vi "Finish.vi"   [LabVIEW 2014]
doc: "This VI is called just before exiting. It is expected to close I/O refnum, save collected data, etc."
uses:
  <vilib>/Rock Robotics/WPI/Joystick/WPI_JoystickGetSetRefNum.vi
  <vilib>/Rock Robotics/WPI/RobotDrive/WPI_RobotDriveGetSetRefNum.vi
  <vilib>/Rock Robotics/WPI/Compressor/WPI_CompressorGetSetRefNum.vi
types:
  T1 = typedef "WPI_CompressorDevRef.ctl" = cluster{"DevStatus":errorcluster, "DigitalInputDevRef":T2, "RelayDevRef":T5}
  T2 = typedef "WPI_DigitalInputDevRef.ctl" = cluster{"DevStatus":errorcluster, "DIO Channel":T3, "Digital Module":T4}
  T3 = typedef "FPGA_DIOChannel.ctl" = enum8{"DIO 1", "DIO 2", "DIO 3", "DIO 4", "DIO 5", "DIO 6", "DIO 7", "DIO 8", "DIO 9", "DIO 10", "DIO 11", "DIO 12", "DIO 13", "DIO 14", "Invalid"}
  T4 = typedef "FPGA_TypedefDigitalModule.ctl" = enum16{"Digital Module 1", "Digital Module 2"}
  T5 = typedef "WPI_RelayDevRef.ctl" = cluster{"DevStatus":errorcluster, "Relay Channel":T6, "Digital Module":T4, "Relay Direction":T7}
  T6 = typedef "FPGA_DIORelayChannel.ctl" = enum8{"Relay 1", "Relay 2", "Relay 3", "Relay 4", "Relay 5", "Relay 6", "Relay 7", "Relay 8", "Invalid"}
  T7 = typedef "WPI_RelayDirection.ctl" = enum16{"Both directions", "Forward only", "Reverse only"}
  T8 = typedef "WPI_CounterDevRef.ctl" = cluster{"DevStatus":errorcluster, "CntIndex":T9}
  T9 = typedef "FPGA_CounterCtrSystemIndex.ctl" = enum8{"Ctr 0", "Ctr 1", "Ctr 2", "Ctr 3", "Ctr 4", "Ctr 5", "Ctr 6", "Ctr 7", "Invalid"}
  T10 = typedef "WPI_EncoderDevRef.ctl" = cluster{"DevStatus":errorcluster, "EncoderIndex":T11, "CounterIndex":T9, "DistancePerCount":dbl, "Decoding Type":T12}
  T11 = typedef "FPGA_EncoderIdx.ctl" = enum8{"Enc 0", "Enc 1", "Enc 2", "Enc 3", "Invalid"}
  T12 = typedef "WPI_EncoderType.ctl" = enum16{"1x", "2x", "4x"}
  T13 = typedef "WPI_RobotDriveDevRef.ctl" = cluster{"DevStatus":errorcluster, "Motors[]":T14[], "Square Inputs":bool, "Max Output":dbl}
  T14 = typedef "WPI_MotorControlDeviceRef.ctl" = cluster{"DeviceStatus":errorcluster, "Type":enum16{"PWM", "CAN"}, "PWM":cluster{"Digital Module":T4, "PWM Channel":T15, "DeadBand":T16}, "CAN":cluster{"Device Number":u8, "Control Mode":T17, "Semaphore":T18, "Max Vout":dbl}, "Invert":bool, "TransformRef":T19, "InvTransformRef":T19}
  T15 = typedef "FPGA_DIOPWMChannel.ctl" = enum8{"PWM 1", "PWM 2", "PWM 3", "PWM 4", "PWM 5", "PWM 6", "PWM 7", "PWM 8", "PWM 9", "PWM 10", "Invalid"}
  T16 = typedef "WPI_PWMDeadband.ctl" = cluster{"Name":string, "maxPositivePwm":i32, "minPositivePwm":i32, "centerPwm":i32, "maxNegativePwm":i32, "minNegativePwm":i32, "angularRange":u16}
  T17 = typedef "WPI_CANJaguar_ControlMode.ctl" = enum8{"Percent VBus", "Current", "Speed", "Position", "Voltage"}
  T18 = typedef "Semaphore RefNum" = refnum<k1>
  T19 = typedef "WPI_PWMTransform_ConPane.ctl" = refnum<vi>
  T20 = typedef "WPI_JoystickDevRef.ctl" = cluster{"Device":T21}
  T21 = typedef "WPI_JoystickDeviceEnum.ctl" = enum16{"USB 0", "USB 1", "USB 2", "USB 3", "USB 4", "USB 5"}
  T22 = typedef "WPI_SolenoidDevRef.ctl" = cluster{"DevStatus":errorcluster, "Solenoid Module":T23, "Forward Solenoid Channel":T24, "Reverse Solenoid Channel":T24}
  T23 = typedef "FPGA_TypedefSolenoidModule.ctl" = enum16{"Solenoid Module 1", "Solenoid Module 2"}
  T24 = typedef "WPI_SolenoidChannel.ctl" = enum8{"Solenoid 1", "Solenoid 2", "Solenoid 3", "Solenoid 4", "Solenoid 5", "Solenoid 6", "Solenoid 7", "Solenoid 8", "Invalid"}
  T25 = typedef "WPI_GyroDevRef.ctl" = cluster{"DevStatus":errorcluster, "Analog Module":T26, "Analog Channel":T27, "Offset":dbl, "Gain (VoltsPerDegree/Second)":dbl}
  T26 = typedef "FPGA_TypedefAnalogModule.ctl" = enum16{"Analog Module 1", "Analog Module 2"}
  T27 = typedef "FPGA_AIChannel.ctl" = enum8{"AI 1", "AI 2", "AI 3", "AI 4", "AI 5", "AI 6", "AI 7", "AI 8", "Invalid"}
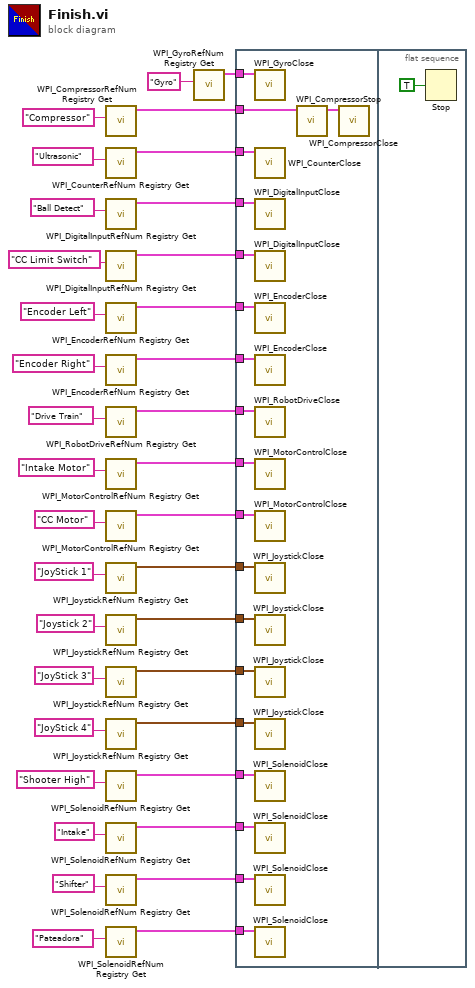
[diagram p0: block diagram]
diagram:
  n1 = call <vilib>:"WPI_CompressorRefNum Registry Get.vi"("refnum name"="Compressor") -> ("CompressorDevRef"=w31:T1)  [unwired: 9 in, 1 out]
  n2 = call <vilib>:"WPI_CounterRefNum Registry Get.vi"("refnum name"="Ultrasonic") -> ("CounterDevRef"=w6:T8)  [unwired: 9 in, 1 out]
  n3 = call <vilib>:"WPI_DigitalInputRefNum Registry Get.vi"("refnum name"="Ball Detect") -> ("DigitalInputDevRef"=w3:T2)  [unwired: 9 in, 1 out]
  n4 = call <vilib>:"WPI_DigitalInputRefNum Registry Get.vi"("refnum name"="CC Limit Switch") -> ("DigitalInputDevRef"=w30:T2)  [unwired: 9 in, 1 out]
  n5 = call <vilib>:"WPI_EncoderRefNum Registry Get.vi"("refnum name"="Encoder Left") -> ("EncoderDevRef"=w1:T10)  [unwired: 9 in, 1 out]
  n6 = call <vilib>:"WPI_EncoderRefNum Registry Get.vi"("refnum name"="Encoder Right") -> ("EncoderDevRef"=w24:T10)  [unwired: 9 in, 1 out]
  n7 = call <vilib>:"WPI_RobotDriveRefNum Registry Get.vi"("refnum name"="Drive Train") -> ("RobotDriveDevRef"=w34:T13)  [unwired: 1 in, 9 out]
  n8 = call <vilib>:"WPI_MotorControlRefNum Registry Get.vi"("refnum name"="Intake Motor") -> ("MotorControlDevRef"=w27:T14)  [unwired: 9 in, 1 out]
  n9 = call <vilib>:"WPI_MotorControlRefNum Registry Get.vi"("refnum name"="CC Motor") -> ("MotorControlDevRef"=w28:T14)  [unwired: 9 in, 1 out]
  n10 = call <vilib>:"WPI_JoystickRefNum Registry Get.vi"("refnum name"="JoyStick 1") -> ("JoystickDevRef"=w12:T20)  [unwired: 9 in, 1 out]
  n11 = call <vilib>:"WPI_JoystickRefNum Registry Get.vi"("refnum name"="Joystick 2") -> ("JoystickDevRef"=w33:T20)  [unwired: 1 in, 9 out]
  n12 = call <vilib>:"WPI_JoystickRefNum Registry Get.vi"("refnum name"="JoyStick 3") -> ("JoystickDevRef"=w10:T20)  [unwired: 9 in, 1 out]
  n13 = call <vilib>:"WPI_JoystickRefNum Registry Get.vi"("refnum name"="JoyStick 4") -> ("JoystickDevRef"=w7:T20)  [unwired: 9 in, 1 out]
  n14 = call <vilib>:"WPI_SolenoidRefNum Registry Get.vi"("refnum name"="Shooter High") -> ("SolenoidDevRef"=w17:T22)  [unwired: 9 in, 1 out]
  n15 = call <vilib>:"WPI_SolenoidRefNum Registry Get.vi"("refnum name"="Intake") -> ("SolenoidDevRef"=w19:T22)  [unwired: 9 in, 1 out]
  n16 = call <vilib>:"WPI_SolenoidRefNum Registry Get.vi"("refnum name"="Shifter") -> ("SolenoidDevRef"=w16:T22)  [unwired: 9 in, 1 out]
  n17 = call <vilib>:"WPI_SolenoidRefNum Registry Get.vi"("refnum name"="Pateadora") -> ("SolenoidDevRef"=w13:T22)  [unwired: 9 in, 1 out]
  n18 = call <vilib>:"WPI_GyroRefNum Registry Get.vi"("refnum name"="Gyro") -> ("GyroDevRef"=w22:T25)  [unwired: 9 in, 1 out]
  n19 = flat-sequence {
    tunnel: w34 -> [w55]
    tunnel: w33 -> [w54]
    tunnel: w31 -> [w53]
    tunnel: w30 -> [w51]
    tunnel: w28 -> [w50]
    tunnel: w27 -> [w49]
    tunnel: w24 -> [w48]
    tunnel: w22 -> [w47]
    tunnel: w19 -> [w46]
    tunnel: w17 -> [w45]
    tunnel: w16 -> [w44]
    tunnel: w13 -> [w43]
    tunnel: w12 -> [w42]
    tunnel: w10 -> [w41]
    tunnel: w7 -> [w40]
    tunnel: w6 -> [w39]
    tunnel: w3 -> [w38]
    tunnel: w1 -> [w37]
    frame #0 {
      n20 = call <vilib>:"WPI_GyroClose.vi"("GyroDevRef"=w47) -> ()  [unwired: 10 in, 1 out]
      n21 = call <vilib>:"WPI_CounterClose.vi"("CounterDevRef"=w39) -> ()  [unwired: 10 in, 1 out]
      n22 = call <vilib>:"WPI_DigitalInputClose.vi"("DigitalInputDevRef"=w38) -> ()  [unwired: 10 in, 1 out]
      n23 = call <vilib>:"WPI_DigitalInputClose.vi"("DigitalInputDevRef"=w51) -> ()  [unwired: 10 in, 1 out]
      n24 = call <vilib>:"WPI_EncoderClose.vi"("EncoderDevRef"=w37) -> ()  [unwired: 10 in, 1 out]
      n25 = call <vilib>:"WPI_EncoderClose.vi"("EncoderDevRef"=w48) -> ()  [unwired: 10 in, 1 out]
      n26 = call <vilib>:"WPI_RobotDriveClose.vi"("RobotDriveDevRef"=w55) -> ()  [unwired: 1 in, 10 out]
      n27 = call <vilib>:"WPI_MotorControlClose.vi"("MotorControlDevRef"=w49) -> ()  [unwired: 10 in, 1 out]
      n28 = call <vilib>:"WPI_MotorControlClose.vi"("MotorControlDevRef"=w50) -> ()  [unwired: 10 in, 1 out]
      n29 = call <vilib>:"WPI_JoystickClose.vi"("JoystickDevRef"=w42) -> ()  [unwired: 11 in]
      n30 = call <vilib>:"WPI_JoystickClose.vi"("JoystickDevRef"=w54) -> ()  [unwired: 11 out]
      n31 = call <vilib>:"WPI_JoystickClose.vi"("JoystickDevRef"=w41) -> ()  [unwired: 11 in]
      n32 = call <vilib>:"WPI_JoystickClose.vi"("JoystickDevRef"=w40) -> ()  [unwired: 11 in]
      n33 = call <vilib>:"WPI_SolenoidClose.vi"("SolenoidDevRef"=w45) -> ()  [unwired: 10 in, 1 out]
      n34 = call <vilib>:"WPI_SolenoidClose.vi"("SolenoidDevRef"=w46) -> ()  [unwired: 10 in, 1 out]
      n35 = call <vilib>:"WPI_SolenoidClose.vi"("SolenoidDevRef"=w44) -> ()  [unwired: 10 in, 1 out]
      n36 = call <vilib>:"WPI_SolenoidClose.vi"("SolenoidDevRef"=w43) -> ()  [unwired: 10 in, 1 out]
      n37 = call <vilib>:"WPI_CompressorStop.vi"("CompressorDevRef"=w53) -> ("CompressorDevRef"=w52:T1)  [unwired: 9 in, 1 out]
      n38 = call <vilib>:"WPI_CompressorClose.vi"("CompressorDevRef"=w52) -> ()  [unwired: 10 in, 1 out]
    }
    frame #1 {
      n39 = Stop(stop? (T)=TRUE ("Quit")) -> ()
    }
  }
